vi "质控报警信息存储 (子VI).vi"   [LabVIEW 2016, in "质控单元.lvlib"]
uses:
  <vilib>/ptbypt/NI_PtbyPt.lvlib
types:
  T1 = cluster{"时间标识":timestamp, "设备":string, "日志信息":string, "流程参数":string}
  T2 = cluster{"时间标识":timestamp, "设备":string, "日志信息":string}
  T3 = cluster{"步骤剩余时间":u16, "当前具体步骤":enum16{"加标", "进样", "排液", "搅拌", "定量"}, " 当前流程":enum16{"", "水样流程", "加标流程", "排液流程"}, "当前小步骤数":i8}
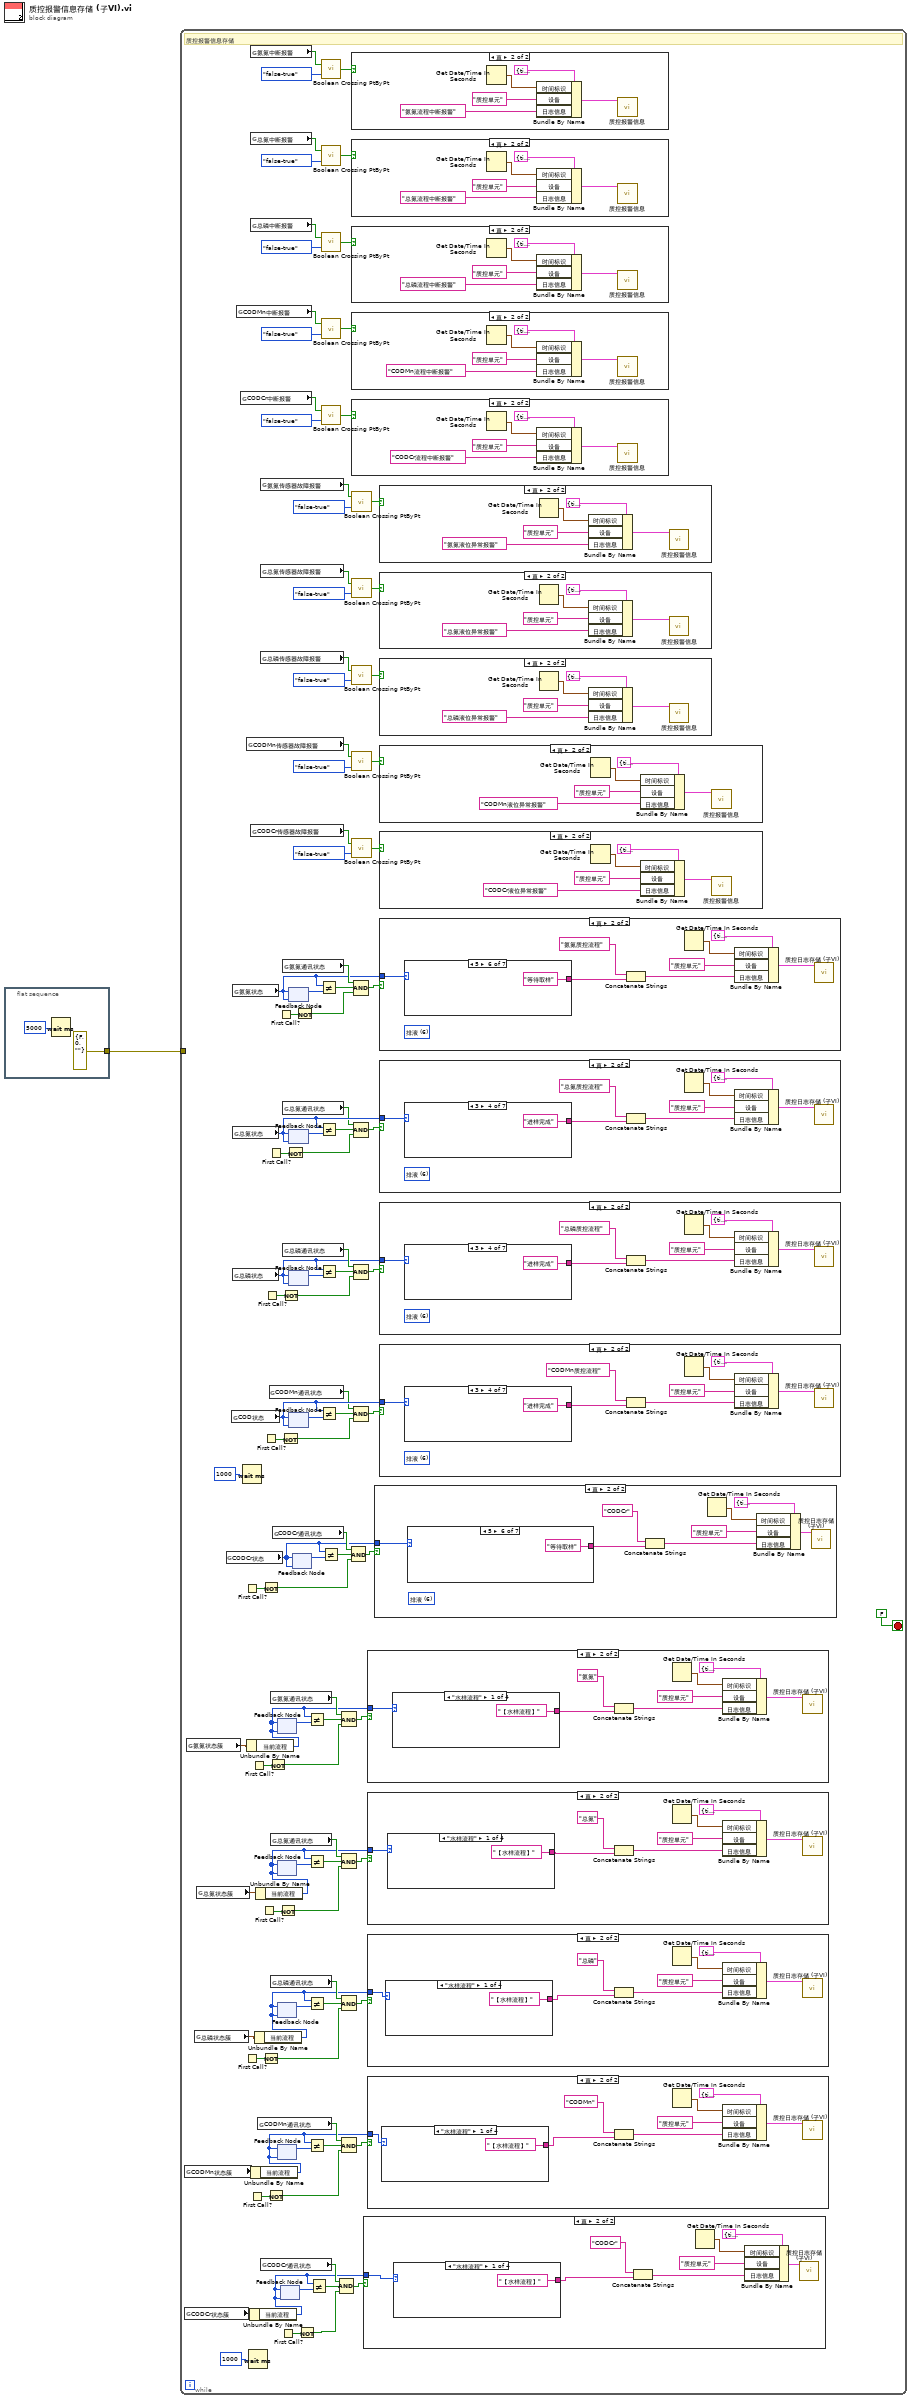
[diagram p0: block diagram]
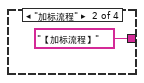
[diagram p3: hidden frame]
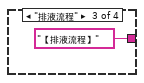
[diagram p4: hidden frame]
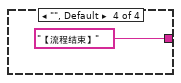
[diagram p5: hidden frame]
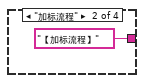
[diagram p7: hidden frame]
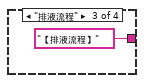
[diagram p8: hidden frame]
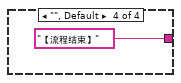
[diagram p9: hidden frame]
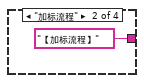
[diagram p11: hidden frame]
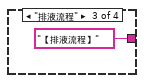
[diagram p12: hidden frame]
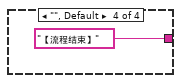
[diagram p13: hidden frame]
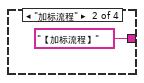
[diagram p15: hidden frame]
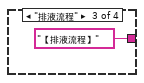
[diagram p16: hidden frame]
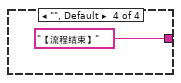
[diagram p17: hidden frame]
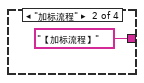
[diagram p19: hidden frame]
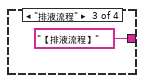
[diagram p20: hidden frame]
diagram:
  n1 = flat-sequence {
    tunnel: [errorcluster {"status"=FALSE, "code"=0, "source"=""} ("错误常量")] -> w1
    frame #0 {
      n2 = Wait (ms)(milliseconds to wait=u32 5000 ("等待时间（毫秒）")) -> ()  [unwired: 1 out]
    }
  }
  n3 = while {
    tunnel: w1 -> [_]
    stop <- FALSE stop-if-true
    # "质控报警信息存储"
    n4 = global read "加标回收状态全局变量.vi" "CODMn状态簇"() -> (w27:T3)
    n5 = global read "加标回收状态全局变量.vi" "CODCr状态簇"() -> (w26:T3)
    n6 = global read "加标回收状态全局变量.vi" "氨氮状态簇"() -> (w33:T3)
    n7 = global read "加标回收状态全局变量.vi" "总磷状态簇"() -> (w29:T3)
    n8 = global read "加标回收状态全局变量.vi" "总氮状态簇"() -> (w31:T3)
    n9 = global read "加标回收状态全局变量.vi" "CODCr状态"() -> (w70:u16)
    n10 = global read "加标回收状态全局变量.vi" "COD状态"() -> (w79:u16)
    n11 = global read "加标回收状态全局变量.vi" "氨氮状态"() -> (w90:u16)
    n12 = global read "加标回收状态全局变量.vi" "总氮状态"() -> (w89:u16)
    n13 = global read "加标回收状态全局变量.vi" "总磷状态"() -> (w80:u16)
    n14 = global read "质控中断报警全局.vi" "CODMn中断报警"() -> (w103:bool)
    n15 = global read "质控中断报警全局.vi" "CODCr中断报警"() -> (w101:bool)
    n16 = Wait (ms)(milliseconds to wait=u32 1000 ("等待时间（毫秒）")) -> ()  [unwired: 1 out]
    n17 = First Call?() -> (First Call?: T/F=w15:bool)
    n18 = First Call?() -> (First Call?: T/F=w9:bool)
    n19 = global read "质控中断报警全局.vi" "CODMn传感器故障报警"() -> (w61:bool)
    n20 = Unbundle By Name(w33) -> ("当前流程"=w32:enum16{"", "水样流程", "加标流程", "排液流程"})
    n21 = First Call?() -> (First Call?: T/F=w7:bool)
    n22 = Wait (ms)(milliseconds to wait=u32 1000 ("等待时间（毫秒）")) -> ()  [unwired: 1 out]
    n23 = First Call?() -> (First Call?: T/F=w13:bool)
    n24 = Unbundle By Name(w26) -> ("当前流程"=w25:enum16{"", "水样流程", "加标流程", "排液流程"})
    n25 = global read "质控中断报警全局.vi" "氨氮中断报警"() -> (w109:bool)
    n26 = global read "质控中断报警全局.vi" "总氮中断报警"() -> (w107:bool)
    n27 = global read "质控中断报警全局.vi" "总磷中断报警"() -> (w105:bool)
    n28 = global read "质控中断报警全局.vi" "CODCr传感器故障报警"() -> (w63:bool)
    n29 = Unbundle By Name(w27) -> ("当前流程"=w24:enum16{"", "水样流程", "加标流程", "排液流程"})
    n30 = Unbundle By Name(w29) -> ("当前流程"=w28:enum16{"", "水样流程", "加标流程", "排液流程"})
    n31 = Unbundle By Name(w31) -> ("当前流程"=w30:enum16{"", "水样流程", "加标流程", "排液流程"})
    n32 = global read "质控内部交互全局.vi" "CODMn通讯状态"() -> (w39:bool)
    n33 = First Call?() -> (First Call?: T/F=w11:bool)
    n34 = global read "质控中断报警全局.vi" "氨氮传感器故障报警"() -> (w55:bool)
    n35 = global read "质控中断报警全局.vi" "总氮传感器故障报警"() -> (w57:bool)
    n36 = global read "质控中断报警全局.vi" "总磷传感器故障报警"() -> (w59:bool)
    n37 = global read "质控内部交互全局.vi" "CODCr通讯状态"() -> (w36:bool)
    n38 = Not(x=w15) -> (.not. x?=w14:bool)
    n39 = Not(x=w9) -> (.not. x?=w8:bool)
    n40 = First Call?() -> (First Call?: T/F=w17:bool)
    n41 = First Call?() -> (First Call?: T/F=w19:bool)
    n42 = Not(x=w7) -> (.not. x?=w6:bool)
    n43 = First Call?() -> (First Call?: T/F=w21:bool)
    n44 = Not(x=w13) -> (.not. x?=w12:bool)
    n45 = global read "质控内部交互全局.vi" "CODMn通讯状态"() -> (w76:bool)
    n46 = global read "质控内部交互全局.vi" "氨氮通讯状态"() -> (w52:bool)
    n47 = global read "质控内部交互全局.vi" "总氮通讯状态"() -> (w47:bool)
    n48 = global read "质控内部交互全局.vi" "总磷通讯状态"() -> (w44:bool)
    n49 = global read "质控内部交互全局.vi" "CODCr通讯状态"() -> (w73:bool)
    n50 = First Call?() -> (First Call?: T/F=w23:bool)
    n51 = feedback #1(w32) -> (w53:enum16{"", "水样流程", "加标流程", "排液流程"})
    n52 = feedback-in #1(w32) -> ()
    n53 = feedback #2(w30) -> (w46:enum16{"", "水样流程", "加标流程", "排液流程"})
    n54 = feedback-in #2(w30) -> ()
    n55 = feedback #3(w28) -> (w45:enum16{"", "水样流程", "加标流程", "排液流程"})
    n56 = feedback-in #3(w28) -> ()
    n57 = feedback #4(w24) -> (w38:enum16{"", "水样流程", "加标流程", "排液流程"})
    n58 = feedback-in #4(w24) -> ()
    n59 = Not(x=w11) -> (.not. x?=w10:bool)
    n60 = First Call?() -> (First Call?: T/F=w5:bool)
    n61 = feedback #5(w25) -> (w37:enum16{"", "水样流程", "加标流程", "排液流程"})
    n62 = feedback-in #5(w25) -> ()
    n63 = Not(x=w17) -> (.not. x?=w16:bool)
    n64 = Not(x=w19) -> (.not. x?=w18:bool)
    n65 = global read "质控内部交互全局.vi" "氨氮通讯状态"() -> (w93:bool)
    n66 = global read "质控内部交互全局.vi" "总氮通讯状态"() -> (w86:bool)
    n67 = global read "质控内部交互全局.vi" "总磷通讯状态"() -> (w83:bool)
    n68 = Not(x=w21) -> (.not. x?=w20:bool)
    n69 = feedback #6(w90) -> (w94:u16)
    n70 = feedback-in #6(w90) -> ()
    n71 = feedback #7(w89) -> (w85:u16)
    n72 = feedback-in #7(w89) -> ()
    n73 = feedback #8(w80) -> (w84:u16)
    n74 = feedback-in #8(w80) -> ()
    n75 = feedback #9(w79) -> (w75:u16)
    n76 = feedback-in #9(w79) -> ()
    n77 = feedback #10(w70) -> (w74:u16)
    n78 = feedback-in #10(w70) -> ()
    n79 = Not(x=w23) -> (.not. x?=w22:bool)
    n80 = Not(x=w5) -> (.not. x?=w4:bool)
    n81 = Not Equal?(x=w32, y=w53) -> (x != y?=w51:bool)
    n82 = Not Equal?(x=w30, y=w46) -> (x != y?=w48:bool)
    n83 = Not Equal?(x=w28, y=w45) -> (x != y?=w43:bool)
    n84 = Not Equal?(x=w24, y=w38) -> (x != y?=w40:bool)
    n85 = Not Equal?(x=w25, y=w37) -> (x != y?=w35:bool)
    n86 = Not Equal?(x=w90, y=w94) -> (x != y?=w92:bool)
    n87 = Not Equal?(x=w89, y=w85) -> (x != y?=w87:bool)
    n88 = Not Equal?(x=w80, y=w84) -> (x != y?=w82:bool)
    n89 = Not Equal?(x=w79, y=w75) -> (x != y?=w77:bool)
    n90 = call <vilib>:"Boolean Crossing PtByPt.vi"("direction"=enum16{"either", "false-true", "true-false"}."false-true", "input"=w109) -> ("crossing"=w99:bool)  [unwired: 1 in]
    n91 = call <vilib>:"Boolean Crossing PtByPt.vi"("direction"=enum16{"either", "false-true", "true-false"}."false-true", "input"=w107) -> ("crossing"=w98:bool)  [unwired: 1 in]
    n92 = call <vilib>:"Boolean Crossing PtByPt.vi"("direction"=enum16{"either", "false-true", "true-false"}."false-true", "input"=w105) -> ("crossing"=w97:bool)  [unwired: 1 in]
    n93 = call <vilib>:"Boolean Crossing PtByPt.vi"("direction"=enum16{"either", "false-true", "true-false"}."false-true", "input"=w103) -> ("crossing"=w96:bool)  [unwired: 1 in]
    n94 = call <vilib>:"Boolean Crossing PtByPt.vi"("direction"=enum16{"either", "false-true", "true-false"}."false-true", "input"=w101) -> ("crossing"=w95:bool)  [unwired: 1 in]
    n95 = Not Equal?(x=w70, y=w74) -> (x != y?=w72:bool)
    n96 = Compound Arithmetic op=AND ("复合运算")(w36, w35, w4) -> (w34:bool)
    n97 = Compound Arithmetic op=AND ("复合运算")(w52, w51, w12) -> (w50:bool)
    n98 = Compound Arithmetic op=AND ("复合运算")(w47, w48, w10) -> (w49:bool)
    n99 = Compound Arithmetic op=AND ("复合运算")(w44, w43, w8) -> (w42:bool)
    n100 = Compound Arithmetic op=AND ("复合运算")(w39, w40, w6) -> (w41:bool)
    n101 = case shown="真" w99 {
      frame False {
      }
      frame True {
        n102 = Get Date/Time In Seconds() -> (seconds since 1Jan1904=w296:timestamp)
        n103 = Bundle By Name(cluster=T2 {"时间标识"=timestamp(0 s since 1904-01-01), "设备"="", "日志信息"=""} ("data in"), "时间标识"=w296, "设备"="质控单元", "日志信息"="氨氮流程中断报警") -> (w292:T2)
        n104 = call "质控报警信息.vi"("data in"=w292) -> ()  [unwired: 10 in, 1 out]
      }
    }
    n105 = case shown="真" w98 {
      frame False {
      }
      frame True {
        n106 = Get Date/Time In Seconds() -> (seconds since 1Jan1904=w291:timestamp)
        n107 = Bundle By Name(cluster=T2 {"时间标识"=timestamp(0 s since 1904-01-01), "设备"="", "日志信息"=""} ("data in"), "时间标识"=w291, "设备"="质控单元", "日志信息"="总氮流程中断报警") -> (w287:T2)
        n108 = call "质控报警信息.vi"("data in"=w287) -> ()  [unwired: 10 in, 1 out]
      }
    }
    n109 = case shown="真" w97 {
      frame False {
      }
      frame True {
        n110 = Get Date/Time In Seconds() -> (seconds since 1Jan1904=w286:timestamp)
        n111 = Bundle By Name(cluster=T2 {"时间标识"=timestamp(0 s since 1904-01-01), "设备"="", "日志信息"=""} ("data in"), "时间标识"=w286, "设备"="质控单元", "日志信息"="总磷流程中断报警") -> (w282:T2)
        n112 = call "质控报警信息.vi"("data in"=w282) -> ()  [unwired: 10 in, 1 out]
      }
    }
    n113 = case shown="真" w96 {
      frame False {
      }
      frame True {
        n114 = Get Date/Time In Seconds() -> (seconds since 1Jan1904=w281:timestamp)
        n115 = Bundle By Name(cluster=T2 {"时间标识"=timestamp(0 s since 1904-01-01), "设备"="", "日志信息"=""} ("data in"), "时间标识"=w281, "设备"="质控单元", "日志信息"="CODMn流程中断报警") -> (w277:T2)
        n116 = call "质控报警信息.vi"("data in"=w277) -> ()  [unwired: 10 in, 1 out]
      }
    }
    n117 = case shown="真" w95 {
      frame False {
      }
      frame True {
        n118 = Get Date/Time In Seconds() -> (seconds since 1Jan1904=w276:timestamp)
        n119 = Bundle By Name(cluster=T2 {"时间标识"=timestamp(0 s since 1904-01-01), "设备"="", "日志信息"=""} ("data in"), "时间标识"=w276, "设备"="质控单元", "日志信息"="CODCr流程中断报警") -> (w272:T2)
        n120 = call "质控报警信息.vi"("data in"=w272) -> ()  [unwired: 10 in, 1 out]
      }
    }
    n121 = Compound Arithmetic op=AND ("复合运算")(w73, w72, w14) -> (w71:bool)
    n122 = call <vilib>:"Boolean Crossing PtByPt.vi"("direction"=enum16{"either", "false-true", "true-false"}."false-true", "input"=w55) -> ("crossing"=w65:bool)  [unwired: 1 in]
    n123 = call <vilib>:"Boolean Crossing PtByPt.vi"("direction"=enum16{"either", "false-true", "true-false"}."false-true", "input"=w57) -> ("crossing"=w66:bool)  [unwired: 1 in]
    n124 = call <vilib>:"Boolean Crossing PtByPt.vi"("direction"=enum16{"either", "false-true", "true-false"}."false-true", "input"=w59) -> ("crossing"=w67:bool)  [unwired: 1 in]
    n125 = call <vilib>:"Boolean Crossing PtByPt.vi"("direction"=enum16{"either", "false-true", "true-false"}."false-true", "input"=w61) -> ("crossing"=w68:bool)  [unwired: 1 in]
    n126 = call <vilib>:"Boolean Crossing PtByPt.vi"("direction"=enum16{"either", "false-true", "true-false"}."false-true", "input"=w63) -> ("crossing"=w69:bool)  [unwired: 1 in]
    n127 = Compound Arithmetic op=AND ("复合运算")(w93, w92, w22) -> (w91:bool)
    n128 = Compound Arithmetic op=AND ("复合运算")(w86, w87, w20) -> (w88:bool)
    n129 = Compound Arithmetic op=AND ("复合运算")(w83, w82, w18) -> (w81:bool)
    n130 = Compound Arithmetic op=AND ("复合运算")(w76, w77, w16) -> (w78:bool)
    n131 = case shown="真" w34 {
      tunnel: w25 -> [_ w112]
      frame False {
      }
      frame True {
        n132 = case shown="\"水样流程\"" w112 {
          tunnel: ["【水样流程】" ("日志信息") "【加标流程】" ("日志信息") "【排液流程】" ("日志信息") "【流程结束】" ("日志信息")] -> w113
          frame "水样流程" {
          }
          frame "加标流程" {
          }
          frame "排液流程" {
          }
          frame "", Default {
          }
        }
        n133 = Concatenate Strings("CODCr" ("日志信息"), w113) -> (w114:string)
        n134 = Get Date/Time In Seconds() -> (seconds since 1Jan1904=w117:timestamp)
        n135 = Bundle By Name(cluster=T1 {"时间标识"=timestamp(0 s since 1904-01-01), "设备"="", "日志信息"="", "流程参数"=""} ("data in"), "时间标识"=w117, "设备"="质控单元", "日志信息"=w114) -> (w118:T1)
        n136 = call "质控日志存储 (子VI).vi"("data in"=w118) -> ()  [unwired: 11 in]
      }
    }
    n137 = case shown="真" w50 {
      tunnel: w32 -> [_ w163]
      frame False {
      }
      frame True {
        n138 = case shown="\"水样流程\"" w163 {
          tunnel: ["【水样流程】" ("日志信息") "【加标流程】" ("日志信息") "【排液流程】" ("日志信息") "【流程结束】" ("日志信息")] -> w161
          frame "水样流程" {
          }
          frame "加标流程" {
          }
          frame "排液流程" {
          }
          frame "", Default {
          }
        }
        n139 = Concatenate Strings("氨氮" ("日志信息"), w161) -> (w160:string)
        n140 = Get Date/Time In Seconds() -> (seconds since 1Jan1904=w165:timestamp)
        n141 = Bundle By Name(cluster=T1 {"时间标识"=timestamp(0 s since 1904-01-01), "设备"="", "日志信息"="", "流程参数"=""} ("data in"), "时间标识"=w165, "设备"="质控单元", "日志信息"=w160) -> (w166:T1)
        n142 = call "质控日志存储 (子VI).vi"("data in"=w166) -> ()  [unwired: 11 in]
      }
    }
    n143 = case shown="真" w49 {
      tunnel: w30 -> [_ w149]
      frame False {
      }
      frame True {
        n144 = case shown="\"水样流程\"" w149 {
          tunnel: ["【水样流程】" ("日志信息") "【加标流程】" ("日志信息") "【排液流程】" ("日志信息") "【流程结束】" ("日志信息")] -> w148
          frame "水样流程" {
          }
          frame "加标流程" {
          }
          frame "排液流程" {
          }
          frame "", Default {
          }
        }
        n145 = Concatenate Strings("总氮" ("日志信息"), w148) -> (w150:string)
        n146 = Get Date/Time In Seconds() -> (seconds since 1Jan1904=w153:timestamp)
        n147 = Bundle By Name(cluster=T1 {"时间标识"=timestamp(0 s since 1904-01-01), "设备"="", "日志信息"="", "流程参数"=""} ("data in"), "时间标识"=w153, "设备"="质控单元", "日志信息"=w150) -> (w154:T1)
        n148 = call "质控日志存储 (子VI).vi"("data in"=w154) -> ()  [unwired: 11 in]
      }
    }
    n149 = case shown="真" w42 {
      tunnel: w28 -> [_ w136]
      frame False {
      }
      frame True {
        n150 = case shown="\"水样流程\"" w136 {
          tunnel: ["【水样流程】" ("日志信息") "【加标流程】" ("日志信息") "【排液流程】" ("日志信息") "【流程结束】" ("日志信息")] -> w137
          frame "水样流程" {
          }
          frame "加标流程" {
          }
          frame "排液流程" {
          }
          frame "", Default {
          }
        }
        n151 = Concatenate Strings("总磷" ("日志信息"), w137) -> (w138:string)
        n152 = Get Date/Time In Seconds() -> (seconds since 1Jan1904=w141:timestamp)
        n153 = Bundle By Name(cluster=T1 {"时间标识"=timestamp(0 s since 1904-01-01), "设备"="", "日志信息"="", "流程参数"=""} ("data in"), "时间标识"=w141, "设备"="质控单元", "日志信息"=w138) -> (w142:T1)
        n154 = call "质控日志存储 (子VI).vi"("data in"=w142) -> ()  [unwired: 11 in]
      }
    }
    n155 = case shown="真" w41 {
      tunnel: w24 -> [_ w124]
      frame False {
      }
      frame True {
        n156 = case shown="\"水样流程\"" w124 {
          tunnel: ["【水样流程】" ("日志信息") "【加标流程】" ("日志信息") "【排液流程】" ("日志信息") "【流程结束】" ("日志信息")] -> w125
          frame "水样流程" {
          }
          frame "加标流程" {
          }
          frame "排液流程" {
          }
          frame "", Default {
          }
        }
        n157 = Concatenate Strings("CODMn" ("日志信息"), w125) -> (w126:string)
        n158 = Get Date/Time In Seconds() -> (seconds since 1Jan1904=w129:timestamp)
        n159 = Bundle By Name(cluster=T1 {"时间标识"=timestamp(0 s since 1904-01-01), "设备"="", "日志信息"="", "流程参数"=""} ("data in"), "时间标识"=w129, "设备"="质控单元", "日志信息"=w126) -> (w130:T1)
        n160 = call "质控日志存储 (子VI).vi"("data in"=w130) -> ()  [unwired: 11 in]
      }
    }
    n161 = case shown="真" w71 {
      tunnel: w70 -> [_ w200]
      frame False {
      }
      frame True {
        (unwired) u16 6 items=["待机", "润洗", "进样", "进样完成", "柱塞泵加标", "等待取液", "排液"] ("氨氮状态")
        n162 = case shown="5" w200 {
          tunnel: ["结束" ("日志信息") "润洗" ("日志信息") "进样" ("日志信息") "进样完成" ("日志信息") "柱塞泵加标" ("日志信息") "等待取样" ("日志信息") "排液" ("日志信息")] -> w198
          frame 0, Default {
          }
          frame 1 {
          }
          frame 2 {
          }
          frame 3 {
          }
          frame 4 {
          }
          frame 5 {
          }
          frame 6 {
          }
        }
        n163 = Concatenate Strings("CODCr" ("日志信息"), w198) -> (w197:string)
        n164 = Get Date/Time In Seconds() -> (seconds since 1Jan1904=w202:timestamp)
        n165 = Bundle By Name(cluster=T1 {"时间标识"=timestamp(0 s since 1904-01-01), "设备"="", "日志信息"="", "流程参数"=""} ("data in"), "时间标识"=w202, "设备"="质控单元", "日志信息"=w197) -> (w203:T1)
        n166 = call "质控日志存储 (子VI).vi"("data in"=w203) -> ()  [unwired: 11 in]
      }
    }
    n167 = case shown="真" w65 {
      frame False {
      }
      frame True {
        n168 = Get Date/Time In Seconds() -> (seconds since 1Jan1904=w196:timestamp)
        n169 = Bundle By Name(cluster=T2 {"时间标识"=timestamp(0 s since 1904-01-01), "设备"="", "日志信息"=""} ("data in"), "时间标识"=w196, "设备"="质控单元", "日志信息"="氨氮液位异常报警") -> (w192:T2)
        n170 = call "质控报警信息.vi"("data in"=w192) -> ()  [unwired: 10 in, 1 out]
      }
    }
    n171 = case shown="真" w66 {
      frame False {
      }
      frame True {
        n172 = Get Date/Time In Seconds() -> (seconds since 1Jan1904=w191:timestamp)
        n173 = Bundle By Name(cluster=T2 {"时间标识"=timestamp(0 s since 1904-01-01), "设备"="", "日志信息"=""} ("data in"), "时间标识"=w191, "设备"="质控单元", "日志信息"="总氮液位异常报警") -> (w187:T2)
        n174 = call "质控报警信息.vi"("data in"=w187) -> ()  [unwired: 10 in, 1 out]
      }
    }
    n175 = case shown="真" w67 {
      frame False {
      }
      frame True {
        n176 = Get Date/Time In Seconds() -> (seconds since 1Jan1904=w186:timestamp)
        n177 = Bundle By Name(cluster=T2 {"时间标识"=timestamp(0 s since 1904-01-01), "设备"="", "日志信息"=""} ("data in"), "时间标识"=w186, "设备"="质控单元", "日志信息"="总磷液位异常报警") -> (w182:T2)
        n178 = call "质控报警信息.vi"("data in"=w182) -> ()  [unwired: 10 in, 1 out]
      }
    }
    n179 = case shown="真" w68 {
      frame False {
      }
      frame True {
        n180 = Get Date/Time In Seconds() -> (seconds since 1Jan1904=w181:timestamp)
        n181 = Bundle By Name(cluster=T2 {"时间标识"=timestamp(0 s since 1904-01-01), "设备"="", "日志信息"=""} ("data in"), "时间标识"=w181, "设备"="质控单元", "日志信息"="CODMn液位异常报警") -> (w177:T2)
        n182 = call "质控报警信息.vi"("data in"=w177) -> ()  [unwired: 10 in, 1 out]
      }
    }
    n183 = case shown="真" w69 {
      frame False {
      }
      frame True {
        n184 = Get Date/Time In Seconds() -> (seconds since 1Jan1904=w176:timestamp)
        n185 = Bundle By Name(cluster=T2 {"时间标识"=timestamp(0 s since 1904-01-01), "设备"="", "日志信息"=""} ("data in"), "时间标识"=w176, "设备"="质控单元", "日志信息"="CODCr液位异常报警") -> (w172:T2)
        n186 = call "质控报警信息.vi"("data in"=w172) -> ()  [unwired: 10 in, 1 out]
      }
    }
    n187 = case shown="真" w91 {
      tunnel: w90 -> [_ w260]
      frame False {
      }
      frame True {
        (unwired) u16 6 items=["待机", "润洗", "进样", "进样完成", "柱塞泵加标", "等待取液", "排液"] ("氨氮状态")
        n188 = case shown="5" w260 {
          tunnel: ["结束" ("日志信息") "润洗" ("日志信息") "进样" ("日志信息") "进样完成" ("日志信息") "柱塞泵加标" ("日志信息") "等待取样" ("日志信息") "排液" ("日志信息")] -> w258
          frame 0, Default {
          }
          frame 1 {
          }
          frame 2 {
          }
          frame 3 {
          }
          frame 4 {
          }
          frame 5 {
          }
          frame 6 {
          }
        }
        n189 = Concatenate Strings("氨氮质控流程" ("日志信息"), w258) -> (w257:string)
        n190 = Get Date/Time In Seconds() -> (seconds since 1Jan1904=w262:timestamp)
        n191 = Bundle By Name(cluster=T1 {"时间标识"=timestamp(0 s since 1904-01-01), "设备"="", "日志信息"="", "流程参数"=""} ("data in"), "时间标识"=w262, "设备"="质控单元", "日志信息"=w257) -> (w263:T1)
        n192 = call "质控日志存储 (子VI).vi"("data in"=w263) -> ()  [unwired: 11 in]
      }
    }
    n193 = case shown="真" w88 {
      tunnel: w89 -> [_ w245]
      frame False {
      }
      frame True {
        (unwired) u16 6 items=["待机", "润洗", "进样", "进样完成", "柱塞泵加标", "等待取液", "排液"] ("氨氮状态")
        n194 = case shown="3" w245 {
          tunnel: ["结束" ("日志信息") "润洗" ("日志信息") "进样" ("日志信息") "进样完成" ("日志信息") "柱塞泵加标" ("日志信息") "等待取样" ("日志信息") "排液" ("日志信息")] -> w243
          frame 0, Default {
          }
          frame 1 {
          }
          frame 2 {
          }
          frame 3 {
          }
          frame 4 {
          }
          frame 5 {
          }
          frame 6 {
          }
        }
        n195 = Concatenate Strings("总氮质控流程" ("日志信息"), w243) -> (w242:string)
        n196 = Get Date/Time In Seconds() -> (seconds since 1Jan1904=w247:timestamp)
        n197 = Bundle By Name(cluster=T1 {"时间标识"=timestamp(0 s since 1904-01-01), "设备"="", "日志信息"="", "流程参数"=""} ("data in"), "时间标识"=w247, "设备"="质控单元", "日志信息"=w242) -> (w248:T1)
        n198 = call "质控日志存储 (子VI).vi"("data in"=w248) -> ()  [unwired: 11 in]
      }
    }
    n199 = case shown="真" w81 {
      tunnel: w80 -> [_ w230]
      frame False {
      }
      frame True {
        (unwired) u16 6 items=["待机", "润洗", "进样", "进样完成", "柱塞泵加标", "等待取液", "排液"] ("氨氮状态")
        n200 = case shown="3" w230 {
          tunnel: ["结束" ("日志信息") "润洗" ("日志信息") "进样" ("日志信息") "进样完成" ("日志信息") "柱塞泵加标" ("日志信息") "等待取样" ("日志信息") "排液" ("日志信息")] -> w228
          frame 0, Default {
          }
          frame 1 {
          }
          frame 2 {
          }
          frame 3 {
          }
          frame 4 {
          }
          frame 5 {
          }
          frame 6 {
          }
        }
        n201 = Concatenate Strings("总磷质控流程" ("日志信息"), w228) -> (w227:string)
        n202 = Get Date/Time In Seconds() -> (seconds since 1Jan1904=w232:timestamp)
        n203 = Bundle By Name(cluster=T1 {"时间标识"=timestamp(0 s since 1904-01-01), "设备"="", "日志信息"="", "流程参数"=""} ("data in"), "时间标识"=w232, "设备"="质控单元", "日志信息"=w227) -> (w233:T1)
        n204 = call "质控日志存储 (子VI).vi"("data in"=w233) -> ()  [unwired: 11 in]
      }
    }
    n205 = case shown="真" w78 {
      tunnel: w79 -> [_ w215]
      frame False {
      }
      frame True {
        (unwired) u16 6 items=["待机", "润洗", "进样", "进样完成", "柱塞泵加标", "等待取液", "排液"] ("氨氮状态")
        n206 = case shown="3" w215 {
          tunnel: ["结束" ("日志信息") "润洗" ("日志信息") "进样" ("日志信息") "进样完成" ("日志信息") "柱塞泵加标" ("日志信息") "等待取样" ("日志信息") "排液" ("日志信息")] -> w213
          frame 0, Default {
          }
          frame 1 {
          }
          frame 2 {
          }
          frame 3 {
          }
          frame 4 {
          }
          frame 5 {
          }
          frame 6 {
          }
        }
        n207 = Concatenate Strings("CODMn质控流程" ("日志信息"), w213) -> (w212:string)
        n208 = Get Date/Time In Seconds() -> (seconds since 1Jan1904=w217:timestamp)
        n209 = Bundle By Name(cluster=T1 {"时间标识"=timestamp(0 s since 1904-01-01), "设备"="", "日志信息"="", "流程参数"=""} ("data in"), "时间标识"=w217, "设备"="质控单元", "日志信息"=w212) -> (w218:T1)
        n210 = call "质控日志存储 (子VI).vi"("data in"=w218) -> ()  [unwired: 11 in]
      }
    }
  }
